vi "Read DO.vi"(11 "DO in":refnum<class "DO.lvclass">) -> (2 "DO":bool, 3 "DO out":refnum<class "DO.lvclass">)   [LabVIEW 2019, in "DO.lvclass"]
uses:
  DO.lvclass
  DO.lvclass/DO.ctl
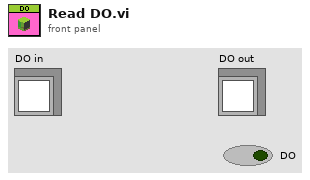
[diagram p1: front panel]
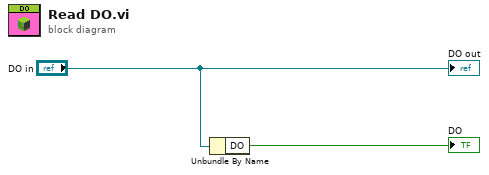
[diagram p0: block diagram]
diagram:
  n1 = Unbundle By Name("DO in") -> ("DO"=→"DO":bool)
  "DO out" <- "DO in"
